vi "Destroy.vi"(0 "reference in":refnum<class "RefferenceA2.lvclass">, 11 "Error In":errorcluster) -> (4 "reference out":refnum<class "RefferenceA2.lvclass">, 15 "Error Out":errorcluster)   [LabVIEW 2018, in "RefferenceA2.lvclass"]
uses:
  RefferenceA2.lvclass
  RefferenceA/RefferenceA.lvclass
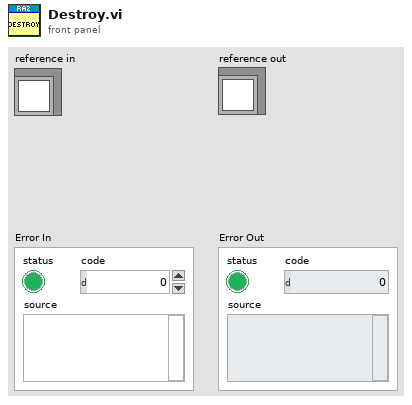
[diagram p1: front panel]
types:
  T1 = typedef "RefferenceA2.lvclass/ObjectAttributes.ctl" = cluster{"Attribute1":dbl}
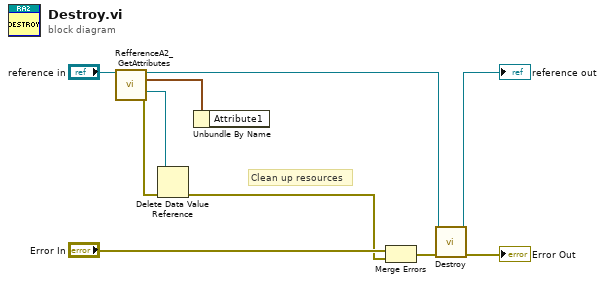
[diagram p0: block diagram]
diagram:
  # "Clean up resources"
  n1 = call "RefferenceA2_GetAttributes.vi"("reference in"="reference in") -> ("reference out"=w3:refnum<class "RefferenceA2.lvclass">, "Data"=w9:T1, "DataRef"=w8:refnum<data-value>, "error out"=w10:errorcluster)  [unwired: 11 in]
  n2 = Delete Data Value Reference(data value reference=w8, error in=w10) -> (error out=w6:errorcluster)  [unwired: 1 out]
  n3 = Unbundle By Name(w9) -> ()  [unwired: 1 out]
  n4 = Merge Errors("Error In", w6) -> (w4:errorcluster)
  n5 = call-parent "Destroy.vi"("reference in"=w3, "Error In"=w4) -> ("reference out"=→"reference out":refnum<class "RefferenceA2.lvclass">, "Error Out"=→"Error Out":errorcluster)  [unwired: 12 in]
